vi "open_path_dialog.vi"(8 "error in":errorcluster, 9 "pattern (all files)":string, 10 "prompt":string) -> (0 "error out":errorcluster, 1 "ok?":bool, 2 "path":path, 4 "exists?":bool)   [LabVIEW 2015]
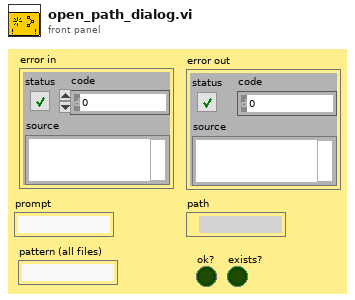
[diagram p1: front panel]
types:
  T1 = enum16{"open", "replace", "create", "open or create", "replace or create", "replace or create with confirmation"}
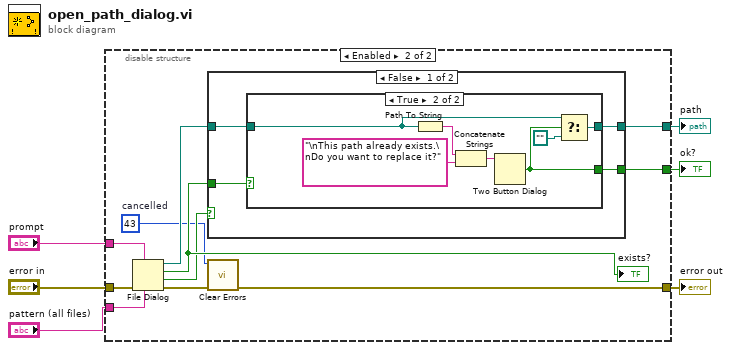
[diagram p0: block diagram]
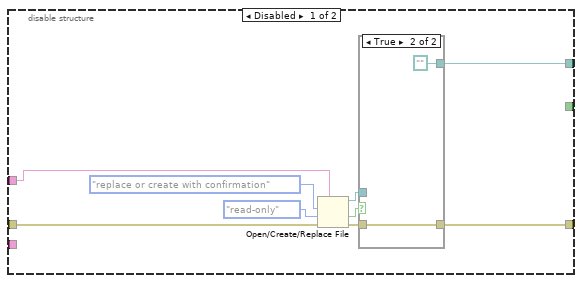
[diagram p2: hidden frame]
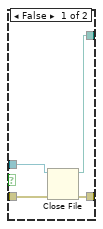
[diagram p3: hidden frame]
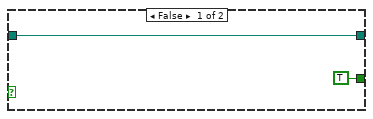
[diagram p4: hidden frame]
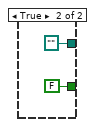
[diagram p5: hidden frame]
diagram:
  n1 = disable-structure shown="Enabled" {
    disable-tunnel: [w12 w28] -> w6
    disable-tunnel: "error in" -> [w9 w31]
    disable-tunnel: [w8 w22] -> w4
    disable-tunnel: "prompt" -> [w7 w32]
    disable-tunnel: [_ w27] -> w2
    disable-tunnel: "pattern (all files)" -> [_ w25]
    frame Disabled {
      n2 = Open/Create/Replace File(error in=w9, prompt=w7, operation (0:open)=T1."replace or create with confirmation", access (0:read/write)=enum16{"read/write", "read-only", "write-only"}."read-only") -> (refnum out=w13:refnum<file>, cancelled=w10:bool, error out=w11:errorcluster)  [unwired: 2 in]
      n3 = case shown="True" w10 {
        tunnel: w13 -> [w19 _]
        tunnel: [w18 path ""] -> w12
        tunnel: w11 -> [w17 w20]
        tunnel: [w16 w20] -> w8
        frame False {
          n4 = Close File(refnum=w19, error in=w17) -> (path=w18:path, error out=w16:errorcluster)
        }
        frame True {
        }
      }
    }
    frame Enabled {
      w24 = 43  # cancelled
      n5 = File Dialog(6:w25, 7:w32, 8:w31) -> (0:w23:errorcluster, 1:w26:bool, 2:w30:bool, 3:w29:path)  [unwired: 4 in]
      "exists?" <- w30
      n6 = case shown="False" w26 {
        tunnel: w30 -> [w36 _]
        tunnel: w29 -> [w35 _]
        tunnel: [w34 path ""] -> w28
        tunnel: [w33 FALSE] -> w27
        frame False {
          n7 = case shown="True" w36 {
            tunnel: w35 -> [w38 w42]
            tunnel: [w38 w40] -> w34
            tunnel: [TRUE w39] -> w33
            frame False {
            }
            frame True {
              n8 = Path To String(path=w42) -> (string=w45:string)
              n9 = Concatenate Strings(w45, "\nThis path already exists.\nDo you want to replace it?" ("message")) -> (w43:string)
              n10 = Two Button Dialog(message=w43) -> (T button?=w39:bool)  [unwired: 2 in]
              n11 = Select(t=w42, s=w39, f=path "") -> (s? t:f=w40:path)
            }
          }
        }
        frame True {
        }
      }
      n12 = call <vilib>:"Clear Errors.vi"("error in (no error)"=w23, "specific error code to clear (0: all)"=w24) -> ("error out"=w22:errorcluster)  [unwired: 4 in, 1 out]
    }
  }
  "path" <- w6
  "error out" <- w4
  "ok?" <- w2
